vi "Climbing to Second Level.vi"(1 "Open arms":bool, 2 "pull wire":bool, 3 "Second Preperation":bool, 4 "close arms":bool) -> (0 "Prep 2":bool)   [LabVIEW 2012]
uses:
  <vilib>/Rock Robotics/WPI/PWM/Servo/WPI_ServoDeviceRef.ctl
  <vilib>/Rock Robotics/SystemInterfaces/Typedef/FPGA_TypedefDigitalModule.ctl
  <vilib>/Rock Robotics/SystemInterfaces/DIO/FPGA_DIOPWMChannel.ctl
  <vilib>/Rock Robotics/WPI/PWM/WPI_PWMDeadband.ctl
  <vilib>/Rock Robotics/WPI/MotorControl/WPI_MotorControlDeviceRef.ctl
  <vilib>/Rock Robotics/WPI/CAN/Jaguar/SubVIs/WPI_CANJaguar_ControlMode.ctl
  <vilib>/Rock Robotics/WPI/PWM/WPI_PWMTransform_ConPane.ctl
  BotStatus.vi
  Motors Values.vi
panel:
  in  "Climbing":bool
  out "Telescopic Arms":dbl
  out "Canenet":dbl
  out "Climbing Enabled?":bool
  in  "Stop Climbing Override":bool
  in  "MotorControlDevRef 2":T1={"DeviceStatus"={"status"=FALSE, "code"=0, "source"=""}, "Type"=enum."PWM", "PWM"={"Digital Module"=enum."Digital Module 1", "PWM Channel"=enum."Invalid", "DeadBand"={"Name"="", "maxPositivePwm"=0, "minPositivePwm"=0, "centerPwm"=0, "maxNegativePwm"=0, "minNegativePwm"=0, "angularRange"=0}}, "CAN"={"Device Number"=0, "Control Mode"=enum."Percent VBus", "Semaphore"=refnum, "Max Vout"=12.0}, "Invert"=FALSE, "TransformRef"=refnum, "InvTransformRef"=refnum}
  in  "MotorControlDevRef 1":T1={"DeviceStatus"={"status"=FALSE, "code"=0, "source"=""}, "Type"=enum."PWM", "PWM"={"Digital Module"=enum."Digital Module 1", "PWM Channel"=enum."Invalid", "DeadBand"={"Name"="", "maxPositivePwm"=0, "minPositivePwm"=0, "centerPwm"=0, "maxNegativePwm"=0, "minNegativePwm"=0, "angularRange"=0}}, "CAN"={"Device Number"=0, "Control Mode"=enum."Percent VBus", "Semaphore"=refnum, "Max Vout"=12.0}, "Invert"=FALSE, "TransformRef"=refnum, "InvTransformRef"=refnum}
  in  "Climbing_ServoDeviceRef":T8={"DeviceStatus"={"status"=FALSE, "code"=0, "source"=""}, "Digital Module"=enum."Digital Module 1", "PWM Channel"=enum."Invalid", "DeadBand"={"Name"="", "maxPositivePwm"=0, "minPositivePwm"=0, "centerPwm"=0, "maxNegativePwm"=0, "minNegativePwm"=0, "angularRange"=0}}
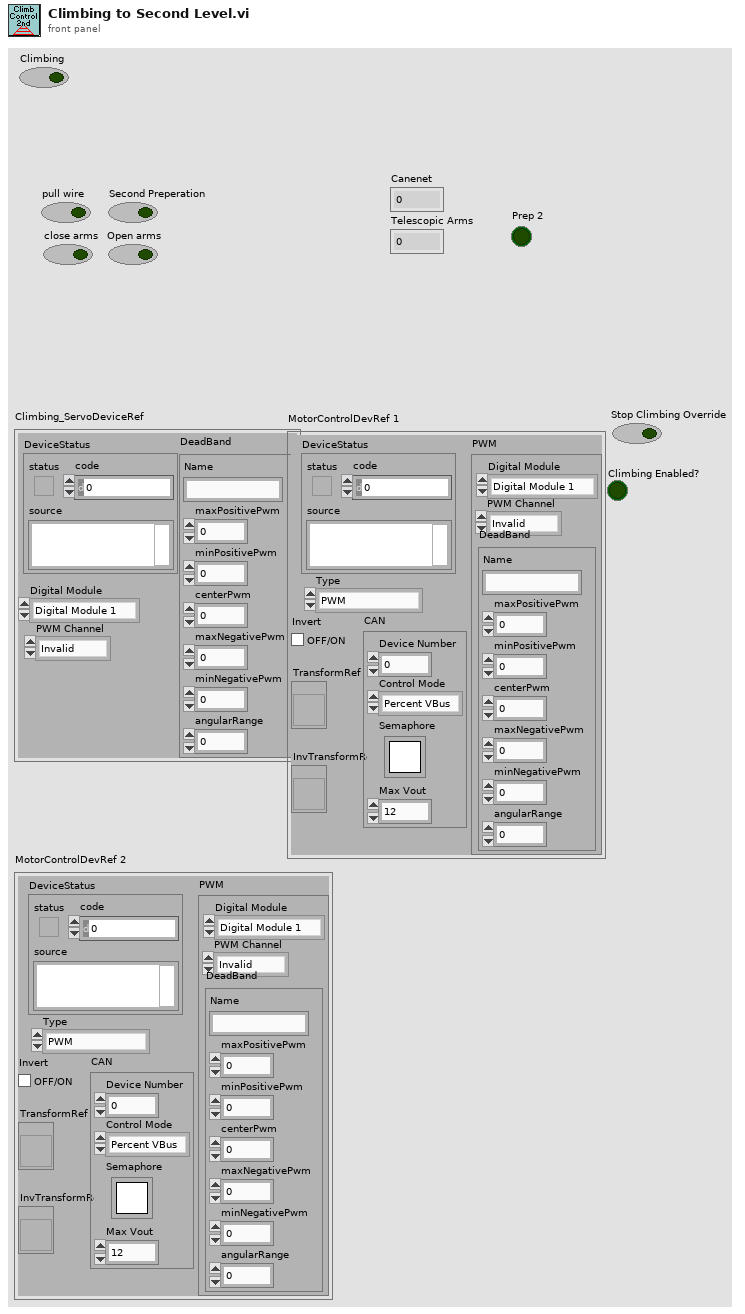
[diagram p1: front panel]
types:
  T1 = typedef "WPI_MotorControlDeviceRef.ctl" = cluster{"DeviceStatus":errorcluster, "Type":enum16{"PWM", "CAN"}, "PWM":cluster{"Digital Module":T2, "PWM Channel":T3, "DeadBand":T4}, "CAN":cluster{"Device Number":u8, "Control Mode":T5, "Semaphore":T6, "Max Vout":dbl}, "Invert":bool, "TransformRef":T7, "InvTransformRef":T7}
  T2 = typedef "FPGA_TypedefDigitalModule.ctl" = enum16{"Digital Module 1", "Digital Module 2"}
  T3 = typedef "FPGA_DIOPWMChannel.ctl" = enum8{"PWM 1", "PWM 2", "PWM 3", "PWM 4", "PWM 5", "PWM 6", "PWM 7", "PWM 8", "PWM 9", "PWM 10", "Invalid"}
  T4 = typedef "WPI_PWMDeadband.ctl" = cluster{"Name":string, "maxPositivePwm":i32, "minPositivePwm":i32, "centerPwm":i32, "maxNegativePwm":i32, "minNegativePwm":i32, "angularRange":u16}
  T5 = typedef "WPI_CANJaguar_ControlMode.ctl" = enum8{"Percent VBus", "Current", "Speed", "Position", "Voltage"}
  T6 = typedef "Semaphore RefNum" = refnum<k1>
  T7 = typedef "WPI_PWMTransform_ConPane.ctl" = refnum<vi>
  T8 = typedef "WPI_ServoDeviceRef.ctl" = cluster{"DeviceStatus":errorcluster, "Digital Module":T2, "PWM Channel":T3, "DeadBand":T4}
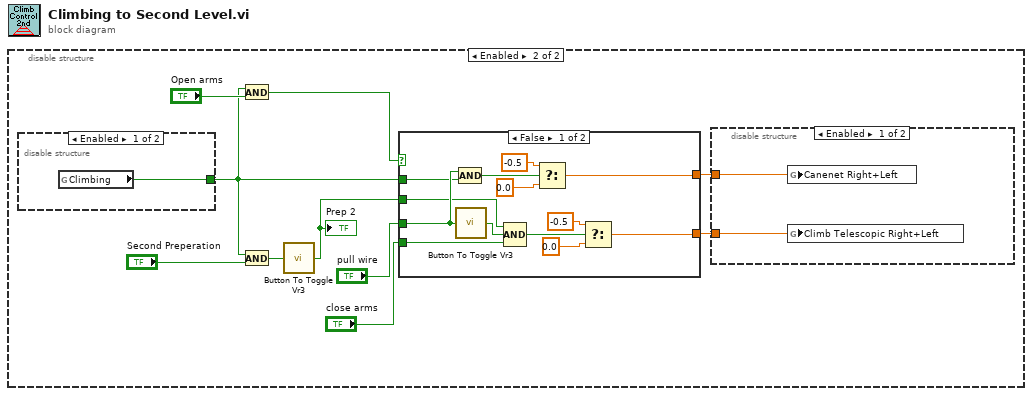
[diagram p0: block diagram]
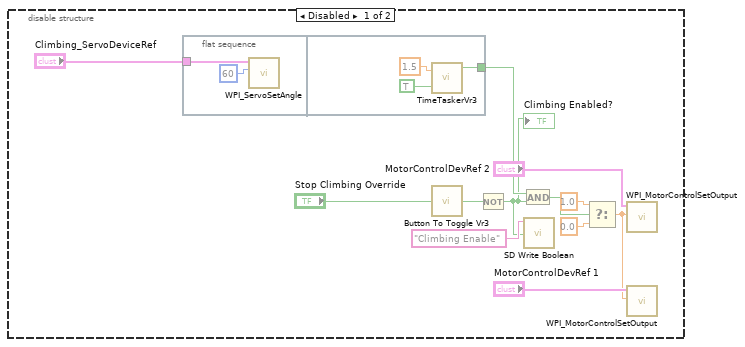
[diagram p2: hidden frame]
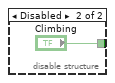
[diagram p3: hidden frame]
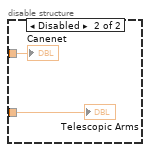
[diagram p4: hidden frame]
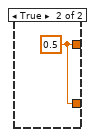
[diagram p5: hidden frame]
diagram:
  n1 = disable-structure shown="Enabled" {
    frame Disabled {
      n2 = flat-sequence {
        tunnel: "Climbing_ServoDeviceRef" -> [w14]
        tunnel: [w16] -> w7
        frame #0 {
          n3 = call <vilib>:"WPI_ServoSetAngle.vi"("Angle"=60, "ServoDeviceRef"=w14) -> ()  [unwired: 8 in, 2 out]
        }
        frame #1 {
          n4 = call "TimeTaskerVr3.vi"("Delay(sec)"=1.5, "Start Counting?"=TRUE) -> ("TimePast?"=w16:bool)  [unwired: 2 out]
        }
      }
      n5 = call "Button To Toggle Vr3.vi"("InValue"="Stop Climbing Override") -> ("Result"=w8:bool)
      n6 = Not(x=w8) -> (.not. x?=w1:bool)
      "Climbing Enabled?" <- w1
      n7 = And(x=w7, y=w1) -> (x .and. y?=w6:bool)
      n8 = call <vilib>:"SD Write Boolean.vi"("Boolean"=w1, "Name"="Climbing Enable") -> ()  [unwired: 8 in, 2 out]
      n9 = Select(t=1.0 ("Delay(sec)"), s=w6, f=0.0 ("Delay(sec)")) -> (s? t:f=w3:dbl)
      n10 = call <vilib>:"WPI_MotorControlSetOutput.vi"("Output"=w3, "MotorControlDevRef"="MotorControlDevRef 2") -> ()  [unwired: 7 in, 3 out]
      n11 = call <vilib>:"WPI_MotorControlSetOutput.vi"("Output"=w3, "MotorControlDevRef"="MotorControlDevRef 1") -> ()  [unwired: 7 in, 3 out]
    }
    frame Enabled {
      n12 = disable-structure shown="Enabled" {
        disable-tunnel: [w28 "Climbing"] -> w23
        frame Enabled {
          n13 = global read "BotStatus.vi" "Climbing"() -> (w28:bool)
        }
        frame Disabled {
        }
      }
      n14 = And(x=w23, y="Open arms") -> (x .and. y?=w27:bool)
      n15 = And(x=w23, y="Second Preperation") -> (x .and. y?=w19:bool)
      n16 = call "Button To Toggle Vr3.vi"("InValue"=w19) -> ("Result"=w18:bool)
      "Prep 2" <- w18
      n17 = case shown="False" w27 {
        tunnel: "close arms" -> [w39 _]
        tunnel: "pull wire" -> [w36 _]
        tunnel: [w42 w47] -> w26
        tunnel: [w41 w47] -> w25
        tunnel: w23 -> [w35 _]
        tunnel: w18 -> [w34 _]
        frame False {
          n18 = call "Button To Toggle Vr3.vi"("InValue"=w36) -> ("Result"=w40:bool)
          n19 = Compound Arithmetic op=AND(w36, w35) -> (w37:bool)
          n20 = Compound Arithmetic op=AND(w34, w40, w39) -> (w38:bool)
          n21 = Select(t=-0.5, s=w37, f=0.0) -> (s? t:f=w42:dbl)
          n22 = Select(t=-0.5, s=w38, f=0.0) -> (s? t:f=w41:dbl)
        }
        frame True {
          w47 = 0.5 ("y")
        }
      }
      n23 = disable-structure shown="Enabled" {
        disable-tunnel: w26 -> [w31 w33]
        disable-tunnel: w25 -> [w30 w32]
        frame Enabled {
          n24 = global write "Motors Values.vi" "Canenet Right+Left"(w31) -> ()
          n25 = global write "Motors Values.vi" "Climb Telescopic Right+Left"(w30) -> ()
        }
        frame Disabled {
          "Canenet" <- w33
          "Telescopic Arms" <- w32
        }
      }
    }
  }
